vi "di5ti.vi"() -> ()   [LabVIEW 2019]
panel:
  out "array 2":dbl[](array[numeric])
  out "array":dbl[][](array[numeric])
  out "String":string
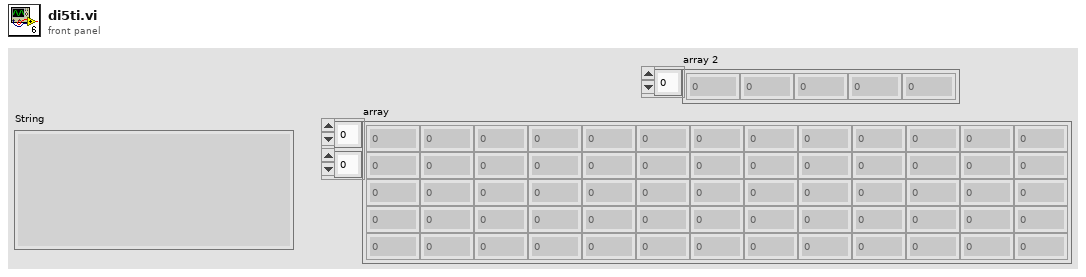
[diagram p1: front panel]
types:
  T1 = enum16{"open", "replace", "create", "open or create", "replace or create", "replace or create with confirmation"}
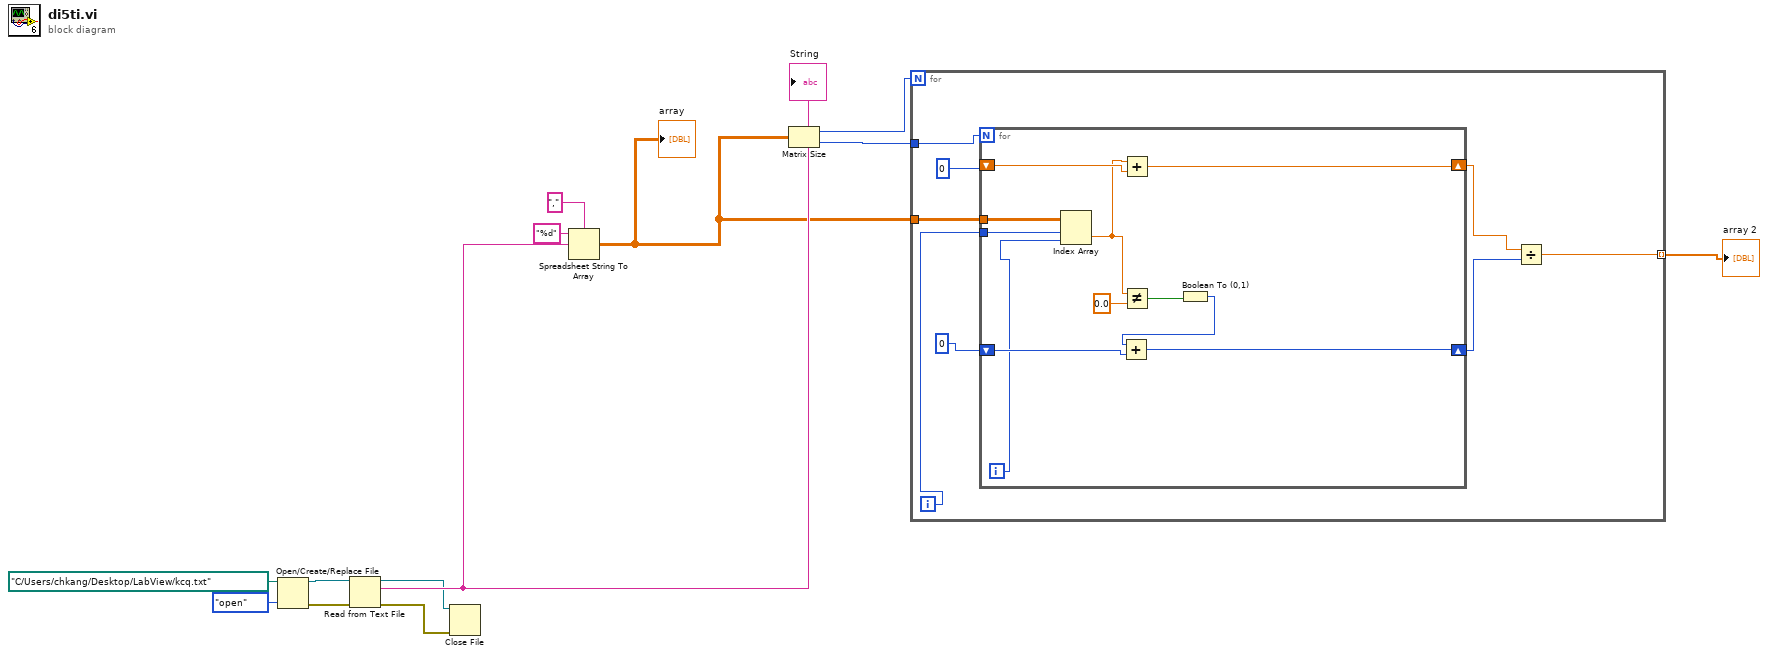
[diagram p0: block diagram]
diagram:
  n1 = Open/Create/Replace File(file path (use dialog)=path "C:/Users/chkang/Desktop/LabView/kcq.txt", operation (0:open)=T1."open") -> (refnum out=w6:refnum<file>, error out=w5:errorcluster)  [unwired: 4 in, 1 out]
  n2 = Read from Text File(file (use dialog)=w6, error in=w5) -> (refnum out=w2:refnum<file>, text=w13:string, error out=w1:errorcluster)  [unwired: 2 in, 1 out]
  "String" <- w13
  n3 = Close File(refnum=w2, error in=w1) -> ()  [unwired: 2 out]
  n4 = Spreadsheet String To Array(delimiter (Tab)=",", format string="%d", spreadsheet string=w13) -> (array=w10:dbl[][])  [unwired: 1 in]
  "array" <- w10
  n5 = Matrix Size(0:w10) -> (1:w8:i32, 2:w7:i32)
  n6 = for {
    N: w8 -> [_]
    tunnel: w10 -> [w21]
    tunnel: [w16] -> w9 mode=indexing
    tunnel: w7 -> [w15]
    i -> [w14]
    n7 = for {
      N: w15 -> [_]
      tunnel: w21 -> [w32]
      shift-right: [w26] -> w18
      shift-left: 0 -> [w25]
      tunnel: w14 -> [w23]
      shift-right: [w27] -> w17
      shift-left: 0 -> [w28]
      i -> [w22]
      n8 = Index Array(array=w32, index (row)=w23, index (col)=w22) -> (element=w24:dbl)
      n9 = Add(x=w24, y=w25) -> (x+y=w26:dbl)
      n10 = Not Equal?(x=w24, y=0.0) -> (x != y?=w30:bool)
      n11 = Boolean To (0,1)(Boolean=w30) -> (0, 1=w29:i16)
      n12 = Add(x=w29, y=w28) -> (x+y=w27:i32)
    }
    n13 = Divide(x=w18, y=w17) -> (x/y=w16:dbl)
  }
  "array 2" <- w9
